vi "Cylinder Display.vi"(8 "error In":errorcluster, 11 "Sequence Context":refnum<k7>) -> (0 "error out":errorcluster)   [LabVIEW 2021, in "OPC UA.lvlib" / "TestExec.lvclass"]
doc: "Use this template to build a simple state machine design pattern. Each state executes code and determines which state to transition to."
uses:
  TestExec.lvclass
  <vilib>/addons/TestStand/_TSUtility.llb/TestStand - Get Property Value (Number {Signed 32-bit Integer}).vi
  <vilib>/addons/TestStand/_TSUtility.llb/TestStand - Get Property Value (Boolean).vi
panel:
  in  "Image Array":string[](array[string])=["Retract All", "DMM Expand", "ACIR Expand", "HiPOT#1 Expand", "HIPOT#2 Expand"]
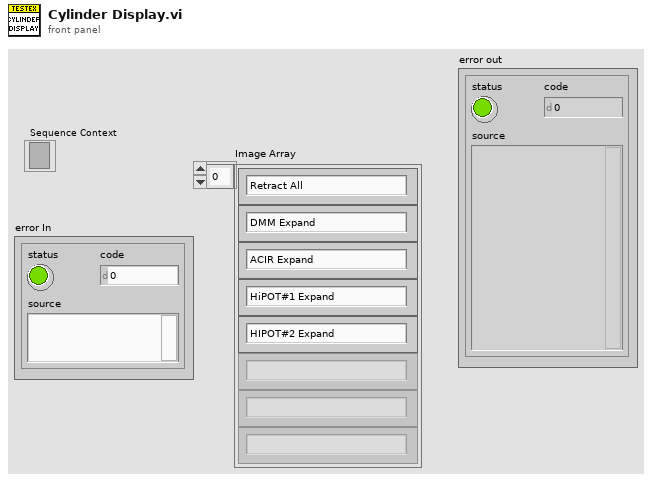
[diagram p1: front panel]
types:
  T1 = typedef "TestStand - Status Monitor.ctl" = cluster{"Sequence Context":refnum<k7>, "Execution":refnum<k7>, "Termination Monitor":refnum<k7>}
  T2 = typedef "imagedata.ctl" = cluster{"image type":i32, "image depth":i32, "image":u8[], "mask":u8[], "colors":u32[], "Rectangle":cluster{"left":i16, "top":i16, "right":i16, "bottom":i16}}
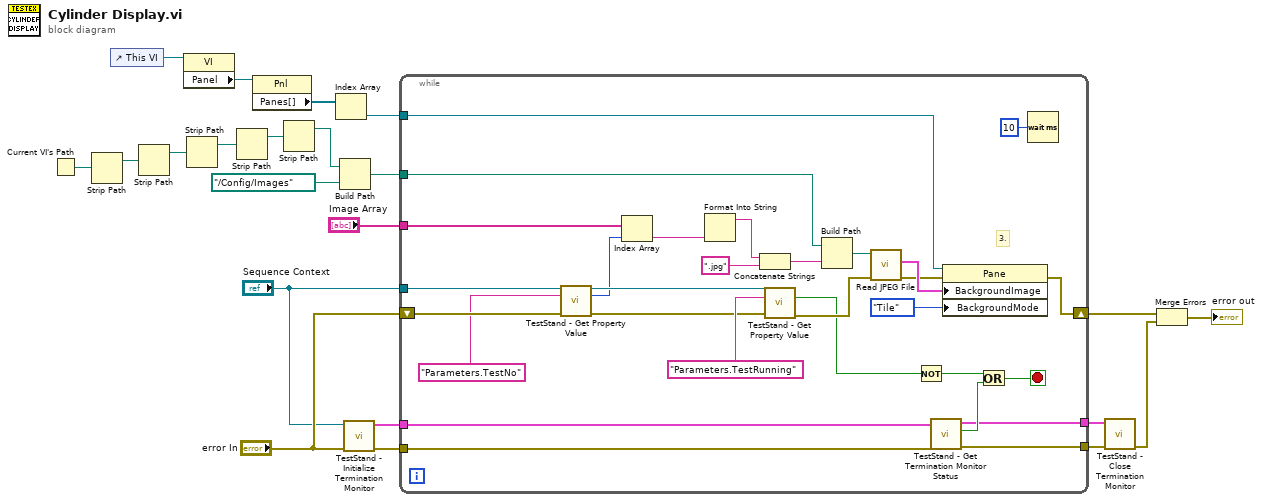
[diagram p0: block diagram]
diagram:
  n1 = Current VI's Path() -> (path=w18:path)
  n2 = Strip Path(path=w18) -> (stripped path=w16:path)  [unwired: 1 out]
  n3 = control-ref of="This VI"() -> (w22:refnum<vi>)
  n4 = Strip Path(path=w16) -> (stripped path=w15:path)  [unwired: 1 out]
  n5 = property class="VI"(reference=w22) -> ("Panel"=w21:refnum<vi>)  [unwired: 1 in, 2 out]
  n6 = Strip Path(path=w15) -> (stripped path=w14:path)  [unwired: 1 out]
  n7 = Strip Path(path=w14) -> (stripped path=w2:path)  [unwired: 1 out]
  n8 = property class="Pnl"(reference=w21) -> ("Panes[]"=w20:refnum<vi>[])  [unwired: 1 in, 2 out]
  n9 = Strip Path(path=w2) -> (stripped path=w1:path)  [unwired: 1 out]
  n10 = Index Array(array=w20) -> (element=w19:refnum<vi>)  [unwired: 1 in]
  n11 = Build Path(base path=w1, name or relative path=path "../Config/Images") -> (appended path=w13:path)
  n12 = call <vilib>:"TestStand - Initialize Termination Monitor.vi"("error in (no error)"="error In", "Sequence Context In"="Sequence Context") -> ("error out"=w8:errorcluster, "Status Monitor Out"=w7:T1)  [unwired: 8 in]
  n13 = while {
    tunnel: w13 -> [w50]
    tunnel: w19 -> [w49]
    shift-right: [w51] -> w12
    shift-left: "error In" -> [w39]
    tunnel: "Image Array" -> [w41]
    tunnel: "Sequence Context" -> [w38]
    tunnel: w8 -> [w30]
    tunnel: w7 -> [w29]
    tunnel: [w26] -> w4
    tunnel: [w25] -> w5
    stop <- w28 stop-if-true
    # "3."
    n14 = call-poly <vilib>:"TestStand - Get Property Value.vi"("Sequence Context In"=w38, "Lookup String"="Parameters.TestNo", "error in (no error)"=w39) -> ("Sequence Context Out"=w36:refnum<k7>, "Value"=w23:i32, "error out"=w34:errorcluster)  [unwired: 10 in]
    n15 = Index Array(array=w41, index=w23) -> (element=w40:string)
    n16 = Format Into String(w40) -> (resulting string=w42:string)  [unwired: 3 in, 1 out]
    n17 = Concatenate Strings(w42, ".jpg" ("string")) -> (w45:string)
    n18 = call-poly <vilib>:"TestStand - Get Property Value.vi"("Sequence Context In"=w36, "Lookup String"="Parameters.TestRunning", "error in (no error)"=w34) -> ("Value"=w32:bool, "error out"=w33:errorcluster)  [unwired: 10 in, 1 out]
    n19 = Build Path(base path=w50, name or relative path=w45) -> (appended path=w48:path)
    n20 = call <vilib>:"Read JPEG File.vi"("error in (no error)"=w33, "path to JPEG file"=w48) -> ("error out"=w43:errorcluster, "image data"=w47:T2)  [unwired: 7 in, 1 out]
    n21 = Not(x=w32) -> (.not. x?=w31:bool)
    n22 = call <vilib>:"TestStand - Get Termination Monitor Status.vi"("error in (no error)"=w30, "Status Monitor In"=w29) -> ("error out"=w26:errorcluster, "Terminating or Aborting"=w27:bool, "Status Monitor Out"=w25:T1)  [unwired: 7 in]
    n23 = property class="Pane"(reference=w49, error in=w43, "BackgroundImage"=w47, "BackgroundMode"=enum16{"Stretch", "Center", "Tile"}."Tile" ("Background Mode")) -> (error out=w51:errorcluster)  [unwired: 1 out]
    n24 = Or(x=w31, y=w27) -> (x .or. y?=w28:bool)
    n25 = Wait (ms)(milliseconds to wait=u32 10) -> ()  [unwired: 1 out]
  }
  n26 = call <vilib>:"TestStand - Close Termination Monitor.vi"("error in (no error)"=w4, "Status Monitor In"=w5) -> ("error out"=w3:errorcluster)  [unwired: 9 in]
  n27 = Merge Errors(w12, w3) -> (→"error out":errorcluster)
